vi "PD(SuppData1)_new.vi"() -> ()   [LabVIEW 2018]
uses:
  <vilib>/Utility/file.llb/Write To Spreadsheet File (DBL).vi
panel:
  in  "Binning factor":i32=1
  in  "Sampling frequency (Hz)":dbl=1000.0
  in  "Stop":bool
  out "Voltage":cluster{dbl[], dbl[]}(graph)
  in  "Save?":bool
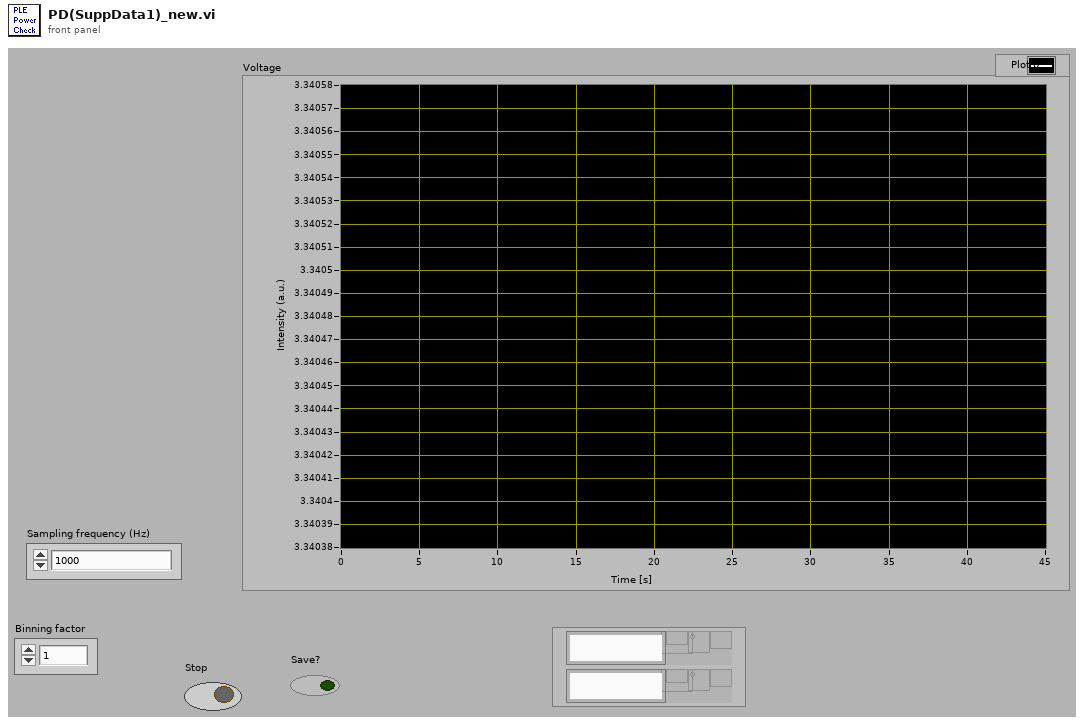
[diagram p1: front panel]
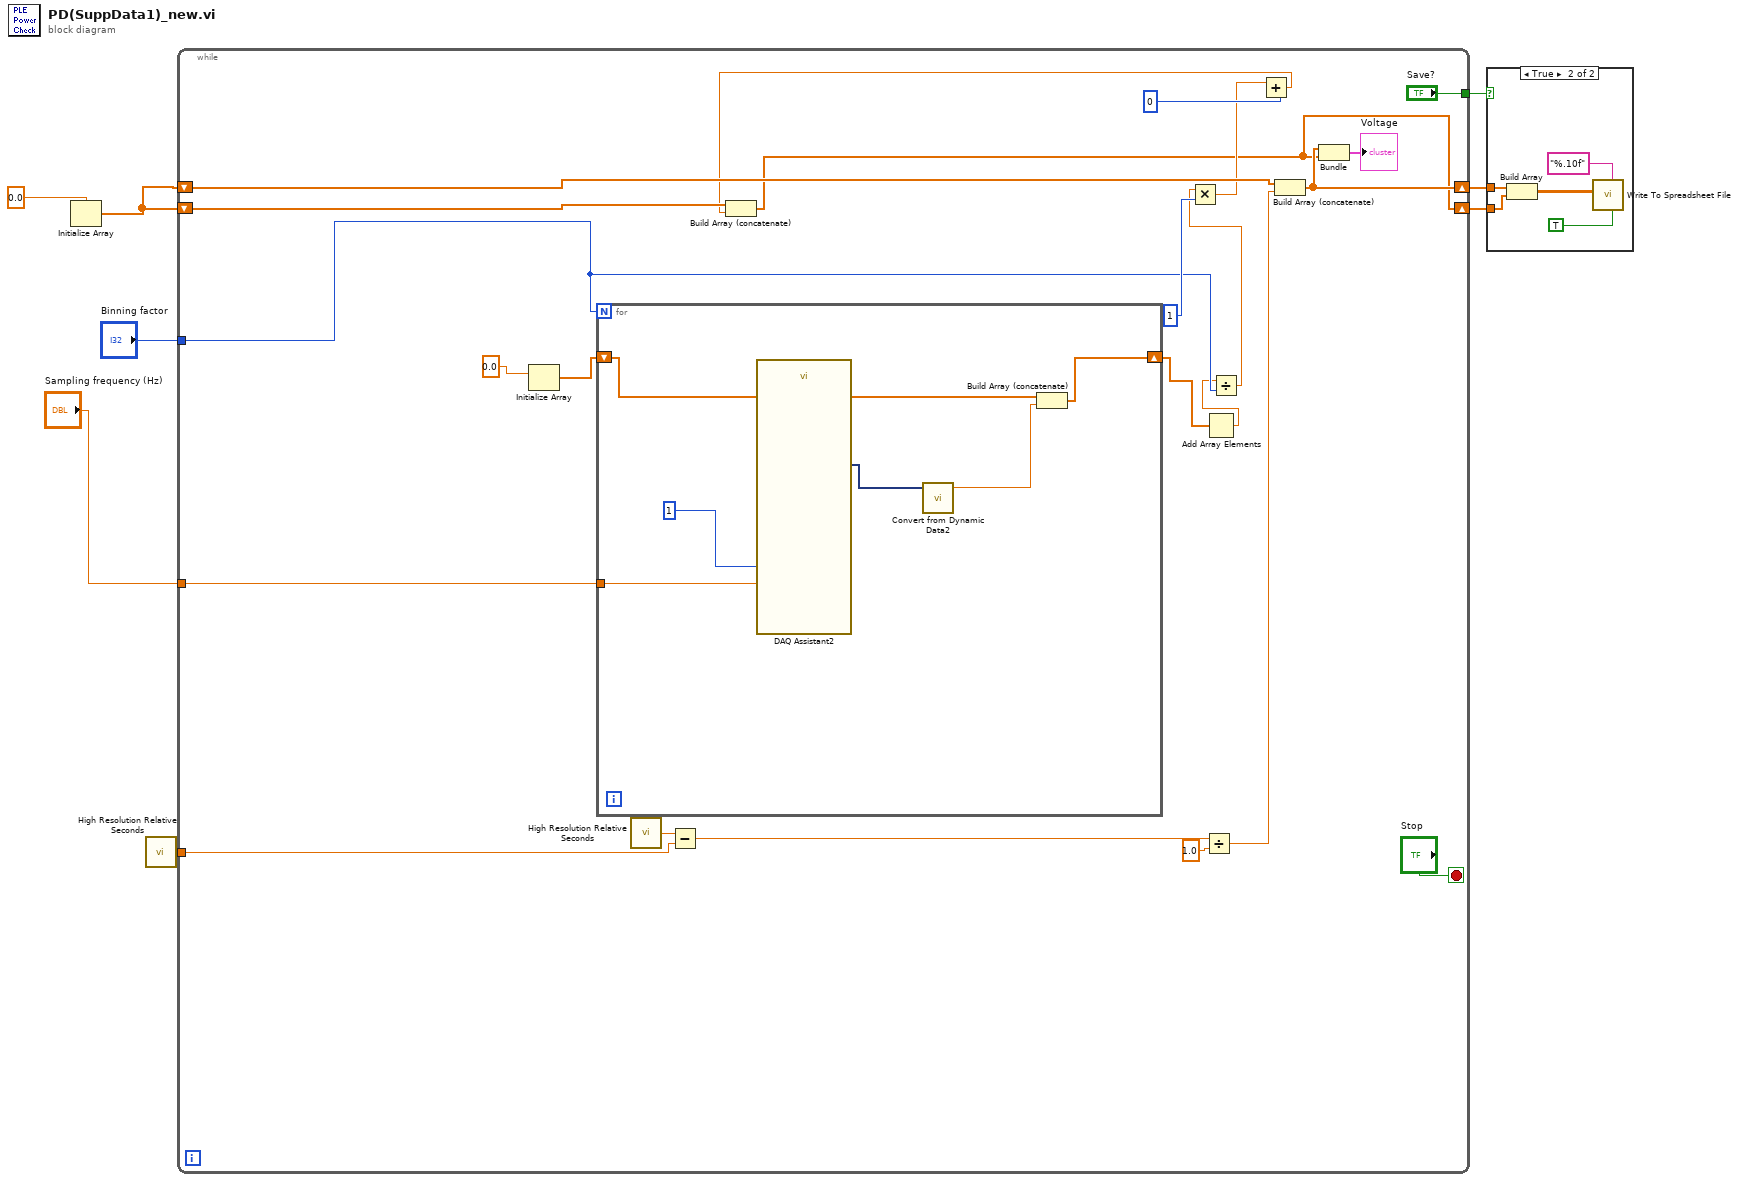
[diagram p0: block diagram]
diagram:
  n1 = Initialize Array(0.0) -> (w1:dbl[])  [unwired: 1 in]
  n2 = call <vilib>:"High Resolution Relative Seconds.vi"() -> ("relative seconds"=w3:dbl)
  n3 = while {
    shift-right: [w9] -> w6
    shift-left: w1 -> [w31]
    shift-right: [w26] -> w5
    shift-left: w1 -> [w30]
    tunnel: "Binning factor" -> [w15]
    tunnel: ["Save?"] -> w4
    tunnel: w3 -> [w23]
    tunnel: "Sampling frequency (Hz)" -> [w17]
    stop <- "Stop" stop-if-true
    n4 = Initialize Array(0.0) -> (w16:dbl[])  [unwired: 1 in]
    n5 = for {
      N: w15 -> [_]
      shift-right: [w33] -> w14
      shift-left: w16 -> [w35]
      tunnel: w17 -> [w37]
      n6 = call "DAQ Assistant2"("rate"=w37, "number of samples"=1) -> ("data"=w36:dynamicdata)  [unwired: 14 in, 3 out]
      n7 = call "Convert from Dynamic Data2"("Dynamic Data Type"=w36) -> ("Scalar"=w34:dbl)  [unwired: 3 in]
      n8 = Build Array (concatenate)(w35, w34) -> (w33:dbl[])
    }
    n9 = call <vilib>:"High Resolution Relative Seconds.vi"() -> ("relative seconds"=w24:dbl)
    n10 = Subtract(x=w24, y=w23) -> (x-y=w22:dbl)
    n11 = Divide(x=w22, y=1.0) -> (x/y=w27:dbl)
    n12 = Add Array Elements(numeric array=w14) -> (sum=w13:dbl)
    n13 = Divide(x=w13, y=w15) -> (x/y=w11:dbl)
    n14 = Multiply(x=w11, y=1) -> (x*y=w19:dbl)
    n15 = Add(x=w19, y=0) -> (x+y=w10:dbl)
    n16 = Build Array (concatenate)(w31, w10) -> (w9:dbl[])
    n17 = Build Array (concatenate)(w30, w27) -> (w26:dbl[])
    n18 = Bundle(w26, w9) -> (→"Voltage":cluster{dbl[], dbl[]})  [unwired: 1 in]
  }
  n19 = case shown="True" w4 {
    tunnel: w6 -> [_ w42]
    tunnel: w5 -> [_ w41]
    frame False {
    }
    frame True {
      n20 = Build Array(w41, w42) -> (w40:dbl[][])
      n21 = call-poly <vilib>:"Write To Spreadsheet File.vi"("transpose? (no:F)"=TRUE, "format (%.3f)"="%.10f", "2D data"=w40) -> ()  [unwired: 5 in, 1 out]
    }
  }
